vi "checksum (SubVI).vi"(11 "incoming data":string="ä¬u\u0003:\u0016 \u0002\u00004d\u001b\u001b\u001b\u00187\u0000\u0000\u000f\u0000\u0000\u0000\u0000\u0000@\u0000\u0000åÿÿÿ^\u000eV\u000eR,\u0013 1627518595.498") -> (1 "CRC matches":bool, 2 "received CRC":u8=19 format="%.0x", 3 "calculated CRC":u8 format="%02x")   [LabVIEW 2018]
panel:
  out "35 bytes":string
  out "35bytes":u8[](array[numeric])=[58, 22, 32, 2, 0, 52, 100, 27, 27, 27, 24, 55, 0, 0, 15, 0, 0, 0, 0, 0, 64, 131, 143, 0, 0, 229, 255, 255, 255, 94, 14, 86, 14, 82, 44] format="%02x"
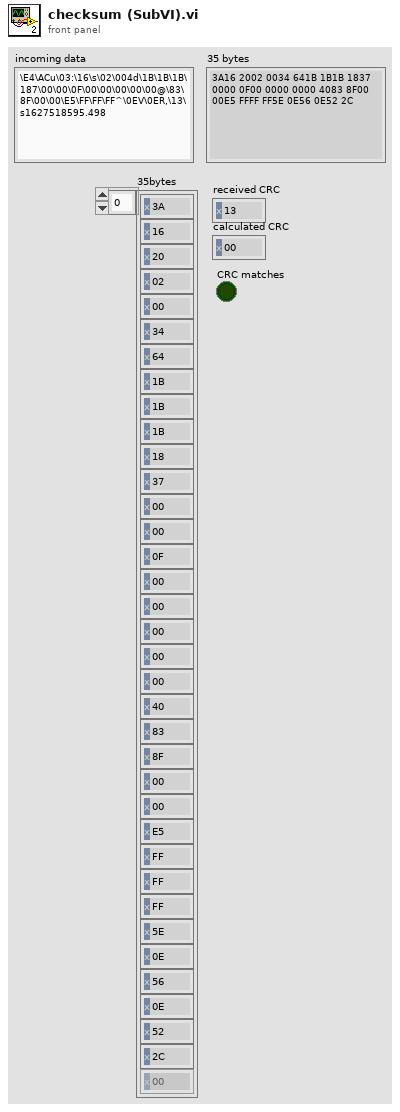
[diagram p1: front panel]
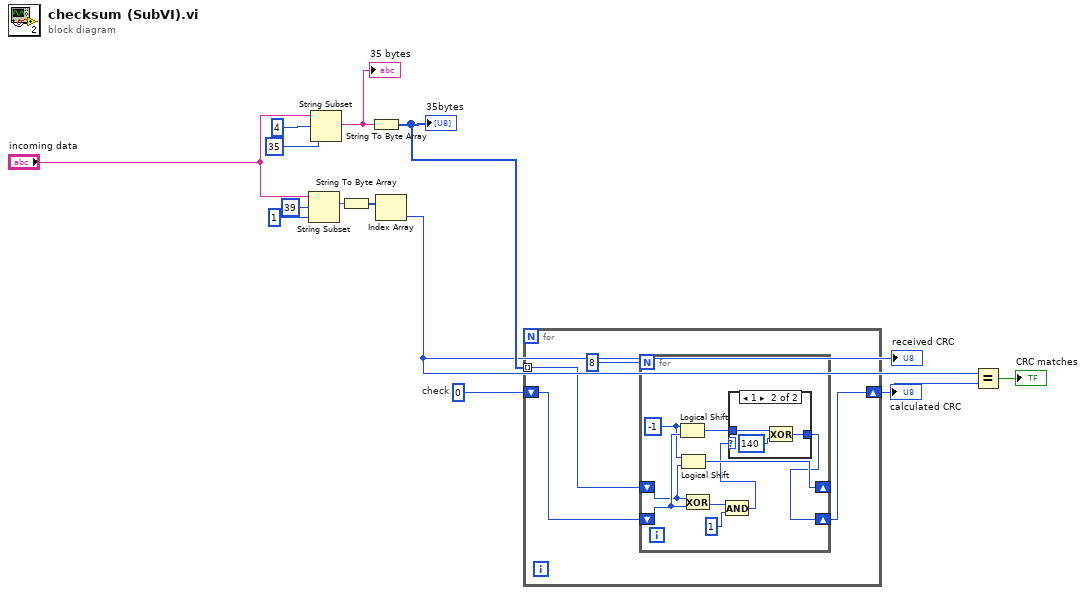
[diagram p0: block diagram]
diagram:
  w4 = u8 0  # check
  n1 = String Subset(string="incoming data", offset (0)=39, length (rest)=1 ("length (rest)")) -> (substring=w9:string)
  n2 = String Subset(string="incoming data", offset (0)=4, length (rest)=35 ("length (rest)")) -> (substring=w6:string)
  "35 bytes" <- w6
  n3 = String To Byte Array(string=w9) -> (unsigned byte array=w8:u8[])
  n4 = String To Byte Array(string=w6) -> (unsigned byte array=w5:u8[])
  "35bytes" <- w5
  n5 = Index Array(array=w8) -> (element=w3:u8)  [unwired: 1 in]
  "received CRC" <- w3
  n6 = for {
    tunnel: w5 -> [w15] mode=indexing
    shift-right: [w14] -> w2
    shift-left: w4 -> [w16]
    n7 = for {
      N: 8 -> [_]
      shift-right: [w18] -> w14
      shift-left: w16 -> [w24]
      shift-right: [w21] -> _
      shift-left: w15 -> [w23]
      w22 = i16 -1 ("y")
      n8 = Logical Shift(y=w22, x=w24) -> (x << y=w19:u8)
      n9 = Logical Shift(y=w22, x=w23) -> (x << y=w21:u8)
      n10 = Exclusive Or(1:w24, 2:w23) -> (0:w26:u8)
      n11 = And(x=w26, y=u8 1) -> (x .and. y?=w20:u8)
      n12 = case shown="1" w20 {
        tunnel: w19 -> [w27 w30]
        tunnel: [w27 w28] -> w18
        frame 0, Default {
        }
        frame 1 {
          n13 = Exclusive Or(1:u8 140 ("y"), 2:w30) -> (0:w28:u8)
        }
      }
    }
  }
  "calculated CRC" <- w2
  n14 = Equal?(x=w3, y=w2) -> (x = y?=→"CRC matches":bool)
